vi "HornScan_SUB_VI.vi"(4 "MessageLength":i32, 5 "Response ID":u8, 6 "Message ID":i32, 7 "error in (no error)":errorcluster, 10 "connection ID":refnum<k5>) -> (0 "error out":errorcluster, 1 "connection ID_out":refnum<k5>, 2 "Resonant Frequencies":string, 3 "Pass":string="Horn Scan Success")   [LabVIEW 2017]
panel:
  # "OUTPUT"
  # "INPUT"
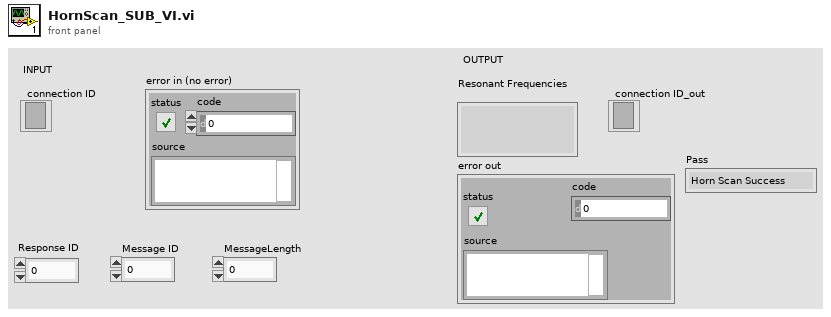
[diagram p1: front panel]
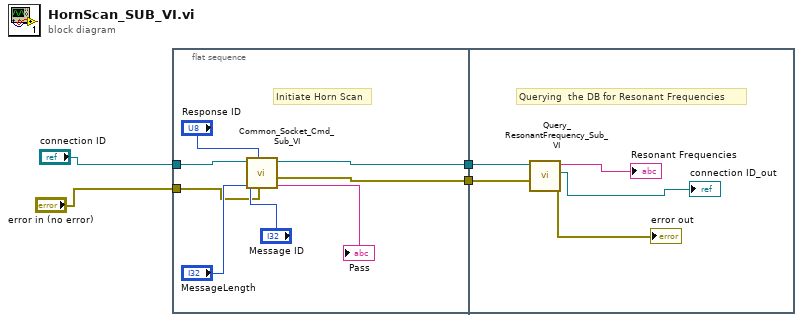
[diagram p0: block diagram]
diagram:
  n1 = flat-sequence {
    tunnel: [w8] -> w4
    tunnel: [w7] -> w3
    tunnel: "connection ID" -> [w6]
    tunnel: "error in (no error)" -> [w5]
    tunnel: w4 -> [w17]
    tunnel: w3 -> [w16]
    frame #0 {
      # "Initiate Horn Scan"
      n2 = call "Common_Socket_Cmd_Sub_VI.vi"("Common Socket Error in"=w5, "Response ID 1"="Response ID", "Operation Message Length 1"="MessageLength", "Operation Message ID 1"="Message ID", "connection ID"=w6) -> ("Status"=→"Pass":string, "error out"=w7:errorcluster, "connection ID"=w8:refnum<k5>)  [unwired: 4 in]
    }
    frame #1 {
      # "Querying  the DB for Resonant Frequencies"
      n3 = call "Query_ResonantFrequency_Sub_VI.vi"("error in (no error)"=w16, "connection ID"=w17) -> ("error out"=→"error out":errorcluster, "connection ID_out"=→"connection ID_out":refnum<k5>, "Resonant Frequencies"=→"Resonant Frequencies":string)  [unwired: 7 in]
    }
  }
